vi "Estructuras.vi"() -> ()   [LabVIEW 2021]
panel:
  in  "stop":bool
  out "Numeric 2":i32
  out "String 3":string
  in  "Boolean":bool
  out "String 2":string
  in  "String":string
  in  "Numeric":dbl
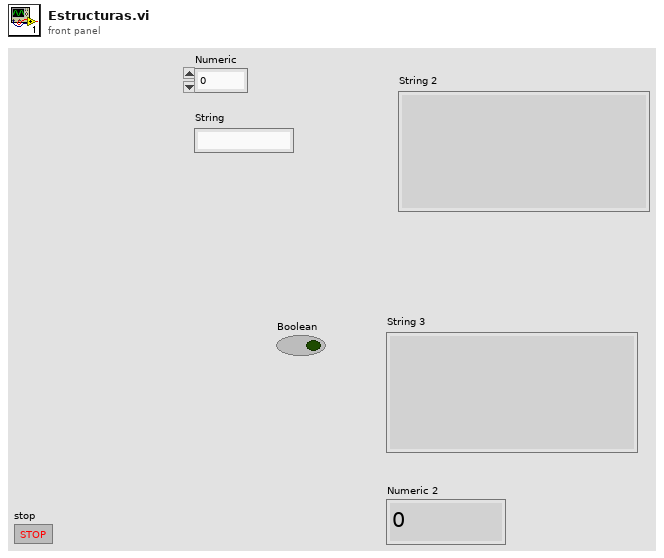
[diagram p1: front panel]
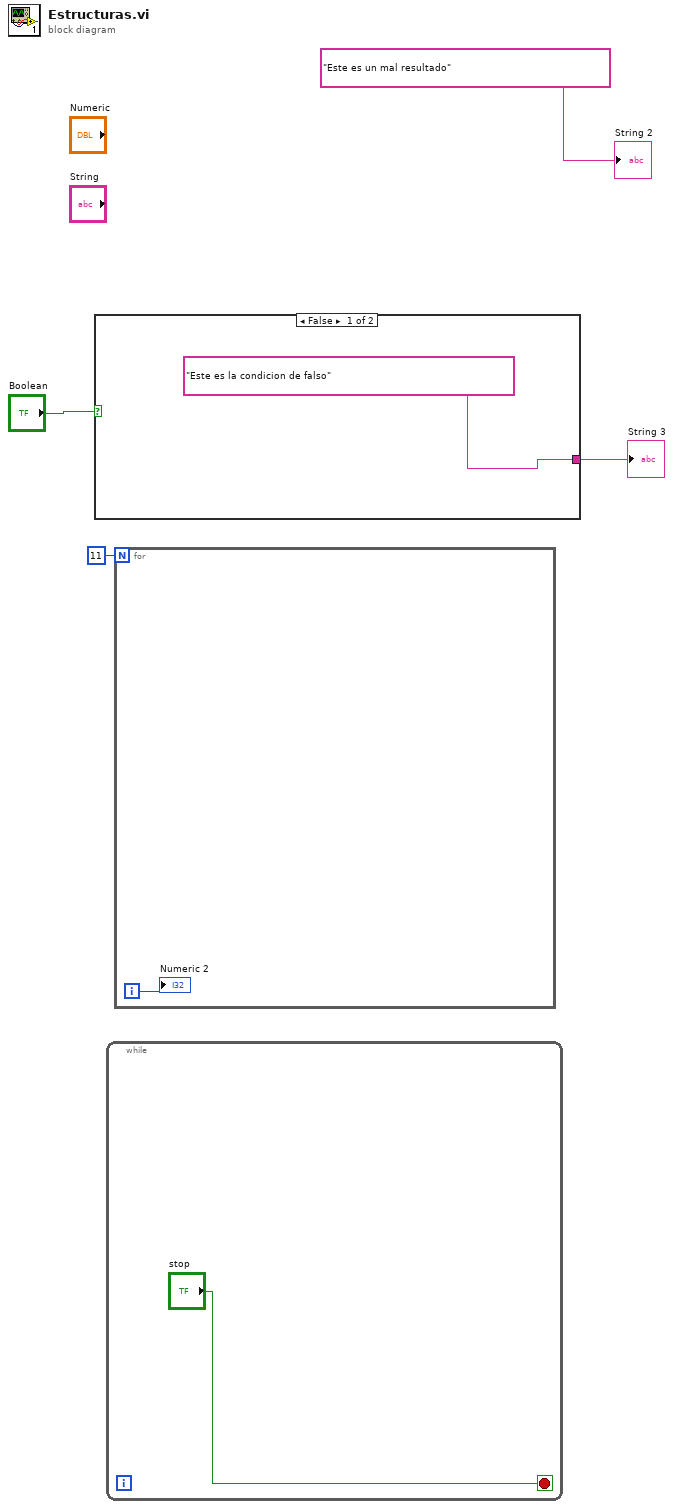
[diagram p0: block diagram]
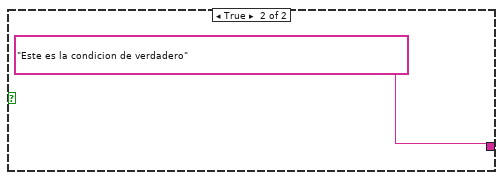
[diagram p2: hidden frame]
diagram:
  n1 = case shown="False" "Boolean" {
    tunnel: ["Este es la condicion de falso" ("String 2") "Este es la condicion de verdadero" ("String 2")] -> w2
    frame False {
    }
    frame True {
    }
  }
  "String 3" <- w2
  n2 = while {
    stop <- "stop" stop-if-true
  }
  n3 = for {
    N: 11 -> [_]
    i -> [w8]
    "Numeric 2" <- w8
  }
  "String 2" <- "Este es un mal resultado" ("String 2")
